vi "Dummy Parms.vi"() -> (0 "I32":i32, 1 "DBL":dbl=3.141592653589793, 2 "path":path, 3 "waveform":waveform(dbl)={"t0"=timestamp(3473168073.631 s since 1904-01-01), "dt"=1e-08, "Y"=[]}, 4 "DBL volts":dbl[unit]=3.141592653589793, 5 "WFG Refnum":refnum<vi>)   [LabVIEW 2010]
panel:
  out "String":string
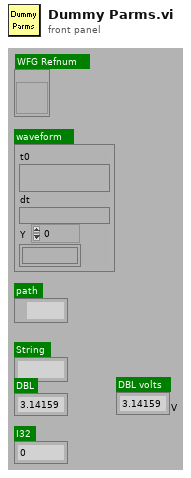
[diagram p1: front panel]
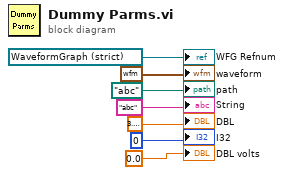
[diagram p0: block diagram]
diagram:
  "WFG Refnum" <- refnum<vi> refnum ("WFG Refnum")
  "waveform" <- waveform(dbl) {"t0"=timestamp(3473168073.631 s since 1904-01-01), "dt"=nan, "Y"=[]} ("waveform")
  "path" <- path "abc" ("path")
  "String" <- "abc" ("String")
  "DBL" <- 3.141592653589793 ("DBL")
  "I32" <- 0 ("I32")
  "DBL volts" <- dbl[unit] 0.0 ("DBL volts")
